vi "Stop piezo.vi"(8 "error in (no error)":errorcluster, 11 "Hardware Configuration":T1) -> (0 "error out":errorcluster)   [LabVIEW 2013, in "Piezo.lvlib"]
uses:
  Piezo/Piezo.lvlib
  Hardware Configuration Piezo.ctl
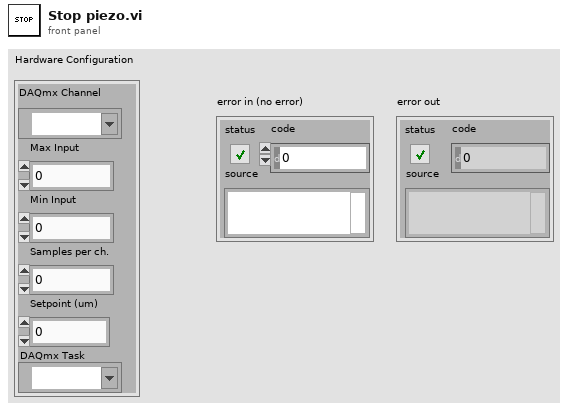
[diagram p1: front panel]
types:
  T1 = typedef "Piezo.lvlib/Hardware Configuration Piezo.ctl" = cluster{"DAQmx Channel":tag, "Max Input":dbl, "Min Input":dbl, "Samples per ch.":dbl, "Setpoint (um)":dbl, "DAQmx Task":refnum<k21>}
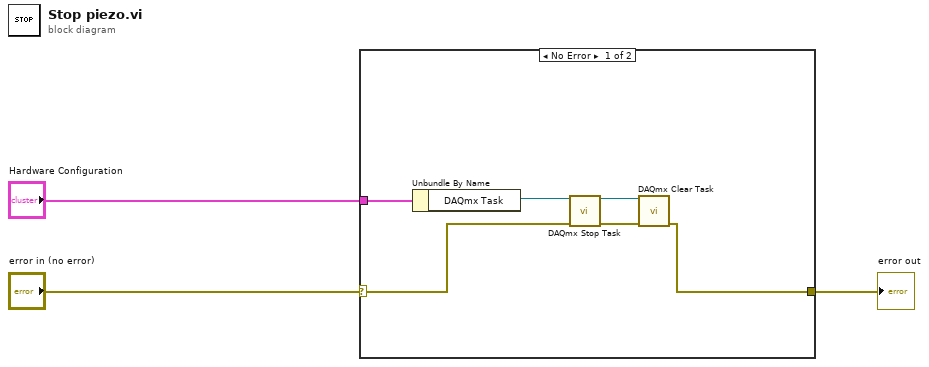
[diagram p0: block diagram]
diagram:
  n1 = case shown="No Error" "error in (no error)" {
    selector: "error in (no error)" -> [w7 w10]
    tunnel: [w4 w10] -> w3
    tunnel: "Hardware Configuration" -> [w9 _]
    frame No Error {
      n2 = Unbundle By Name(w9) -> ("DAQmx Task"=w8:refnum<k21>)
      n3 = call <vilib>:"DAQmx Stop Task.vi"("task/channels in"=w8, "error in"=w7) -> ("task out"=w6:refnum<k21>, "error out"=w5:errorcluster)  [unwired: 12 in]
      n4 = call <vilib>:"DAQmx Clear Task.vi"("task in"=w6, "error in"=w5) -> ("error out"=w4:errorcluster)  [unwired: 13 in]
    }
    frame Error {
    }
  }
  "error out" <- w3
